vi "Parse container ID.vi"(8 "Error In":errorcluster, 10 "\"cmd /c docker ps\" output":string) -> (0 "Error Out":errorcluster, 2 "Firefly iii App Container ID":string)   [LabVIEW 2017]
panel:
  in  "Multicolumn Listbox":i32(listbox)
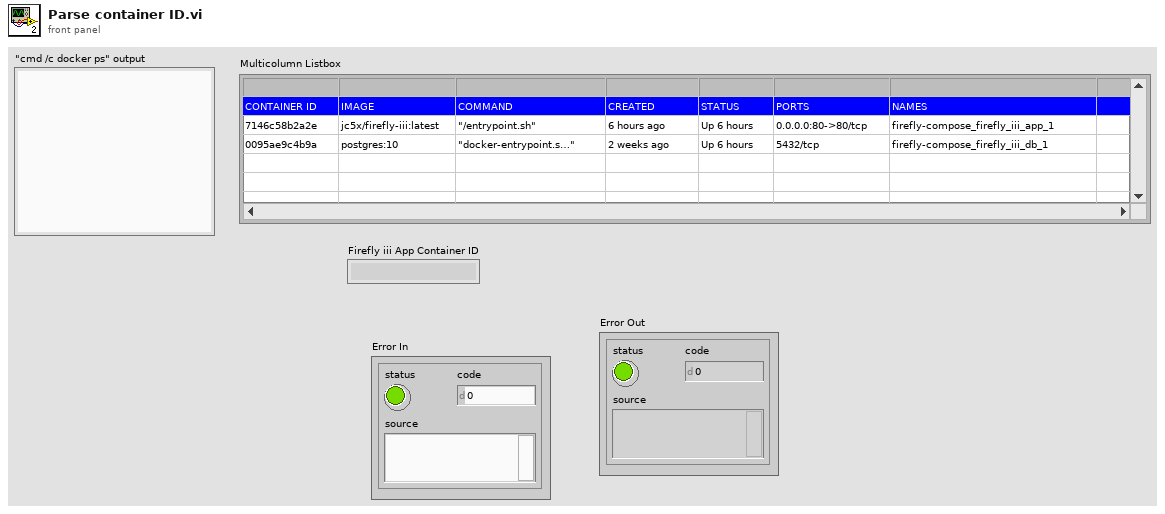
[diagram p1: front panel]
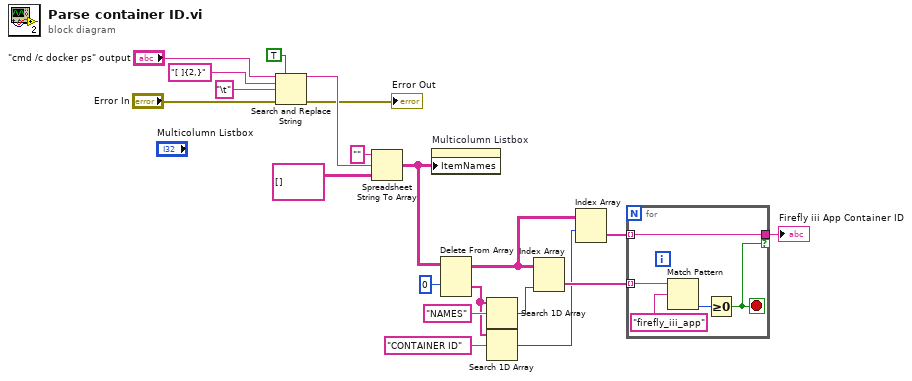
[diagram p0: block diagram]
diagram:
  n1 = Search and Replace String(replace all?=TRUE ("replace all? (F)"), input string="\"cmd /c docker ps\" output", search string="[ ]{2,}", replace string="\t" ("replace string (\"\")"), error in="Error In") -> (result string=w15:string, error out=→"Error Out":errorcluster)  [unwired: 3 in, 2 out]
  n2 = Spreadsheet String To Array(format string="", spreadsheet string=w15, array type (2D Dbl)=string[][] []) -> (array=w13:string[][])  [unwired: 1 in]
  n3 = property on="Multicolumn Listbox" class="MCListbox (strict)"("ItemNames"=w13) -> ()  [unwired: 2 in, 2 out]
  n4 = Delete From Array(array=w13, index (row)=0) -> (deleted portion=w7:string[], array with subset deleted=w6:string[][])  [unwired: 2 in]
  n5 = Search 1D Array(1D array=w7, element="NAMES") -> (index of element=w10:i32)  [unwired: 1 in]
  n6 = Search 1D Array(1D array=w7, element="CONTAINER ID") -> (index of element=w5:i32)  [unwired: 1 in]
  n7 = Index Array(array=w6, index (col)=w10) -> (element=w9:string[])  [unwired: 1 in]
  n8 = Index Array(array=w6, index (row)=w5) -> (element=w4:string[])  [unwired: 1 in]
  n9 = for {
    tunnel: w9 -> [w24] mode=indexing
    tunnel: w4 -> [w22] mode=indexing
    tunnel: [w22] -> w3 if=w21
    stop <- w21 stop-if-true
    n10 = Match Pattern(string=w24, regular expression="firefly_iii_app") -> (offset past match=w23:i32)  [unwired: 1 in, 3 out]
    n11 = Greater Or Equal To 0?(x=w23) -> (x >= 0?=w21:bool)
  }
  "Firefly iii App Container ID" <- w3
